vi "Dispose.vi"(8 "error in":errorcluster, 11 "NYStylePepperoniPizza":refnum<class "NYStylePepperoniPizza.lvclass">) -> (0 "error out":errorcluster)   [LabVIEW 2020, in "FactoryMethod.lvlib" / "PizzaFactoryMethod.lvlib" / "NYStylePepperoniPizza.lvclass"]
uses:
  NYStylePepperoniPizza.lvclass
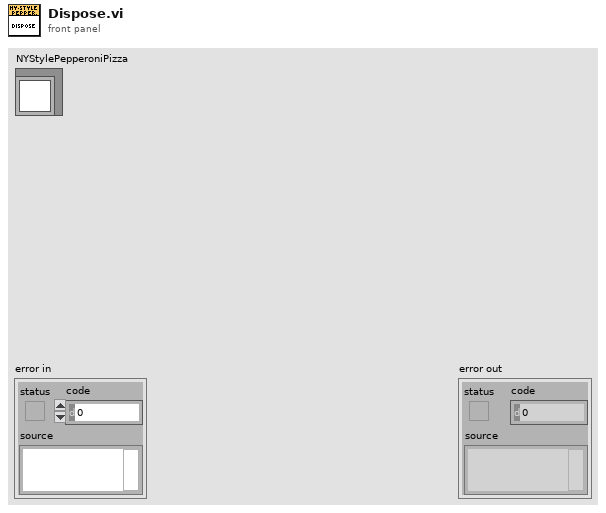
[diagram p1: front panel]
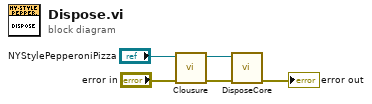
[diagram p0: block diagram]
diagram:
  n1 = call-dynamic "Clousure.vi"("error in"="error in", "NYStylePepperoniPizza"="NYStylePepperoniPizza") -> ("error out"=w3:errorcluster, "NYStylePepperoniPizza"=w4:refnum<class "NYStylePepperoniPizza.lvclass">)  [unwired: 8 in]
  n2 = call-dynamic "DisposeCore.vi"("error in (no error)"=w3, "NYStylePepperoniPizza"=w4) -> ("error out"=→"error out":errorcluster)  [unwired: 8 in, 1 out]
